vi "TEST X Listbox.vi"() -> ()   [LabVIEW 2009]
doc: "This VI is used to test the X Listbox XControl that is developed in the exercise.,\n\nAAL 9/09"
panel:
  out "Deleted Item":string
  out "Invalid Item?":bool
  in  "Delete All":bool
  in  "Item Name":string
  in  "Add Item":bool
  in  "Delete Item":bool
  in  "Delete Item":string
  in  "Exit":bool
  out "X Control Output":string
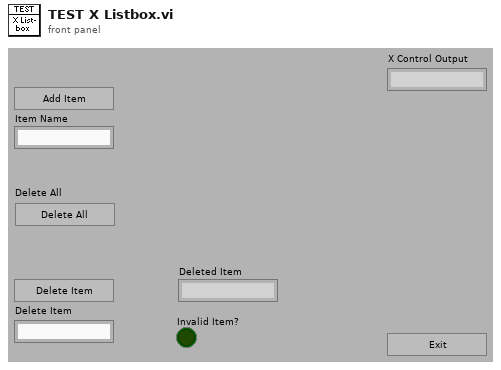
[diagram p1: front panel]
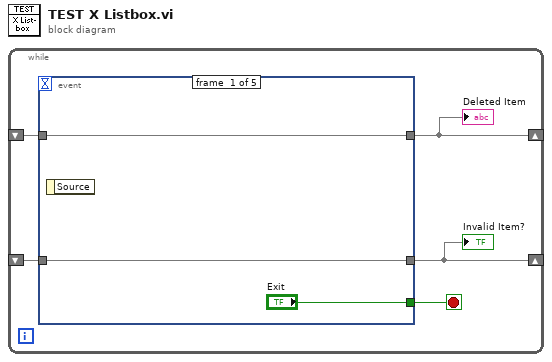
[diagram p0: block diagram]
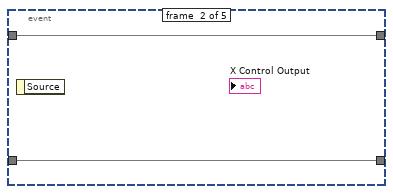
[diagram p2: hidden frame]
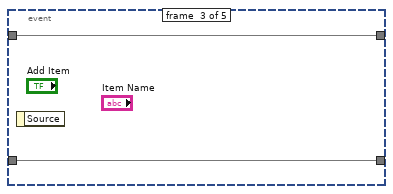
[diagram p3: hidden frame]
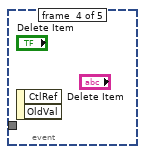
[diagram p4: hidden frame]
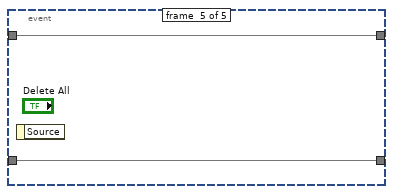
[diagram p5: hidden frame]
diagram:
  n1 = while {
    shift-right: [w4] -> _
    shift-left: _ -> [w3]
    shift-right: [w2] -> _
    shift-left: _ -> [w1]
    stop <- w5 stop-if-true
    n2 = event shown="[4] \"Delete All\": Value Change" {
      selector: _ -> [_ _ _ _ _]
      dyn-events: _ -> [_ _ _ _ _]
      timeout: _ -> [_ _ _ _ _]
      tunnel: ["Exit" _ _ _ _] -> w5
      tunnel: [w6 w9 w11 _ w13] -> w2
      tunnel: [w7 w10 w12 _ w14] -> w4
      tunnel: w3 -> [w7 w10 w12 _ w14]
      tunnel: w1 -> [w6 w9 w11 _ w13]
      event #0 {
        n3 = event-data() -> ()  [unwired: 2 out]
      }
      event #1 {
        n4 = event-data() -> ()  [unwired: 2 out]
      }
      event #2 {
        n5 = event-data() -> ()  [unwired: 2 out]
      }
      event #3 {
        n6 = event-data() -> ()  [unwired: 3 out]
      }
      event #4 {
        n7 = event-data() -> ()  [unwired: 2 out]
      }
    }
    "Invalid Item?" <- w2
    "Deleted Item" <- w4
  }
